vi "Utility Read From Register - Integers.vi"(0 "VISA resource name":refnum<visa-resource-name>, 1 "Unit Address (1)":u8=1, 5 "Register Address (0)":u16, 9 "Num Of Reg (1)":u16=1 min=1 step=1, 11 "error in (no error)":errorcluster) -> (4 "VISA resource name out":refnum<visa-resource-name>, 6 "Data":i16[](array[numeric]), 15 "error out":errorcluster)   [LabVIEW 2010, in "Eurotherm 32xx Series.lvlib"]
doc: "This VI reads value from specified registers of specified unit."
uses:
  <instrlib>/Eurotherm 32xx Series/Eurotherm 32xx Series.lvlib
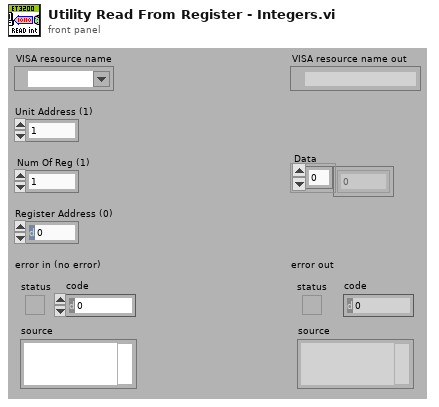
[diagram p1: front panel]
types:
  T1 = cluster{"Read Buffer[0]":u8, "Read Buffer[1]":u8}
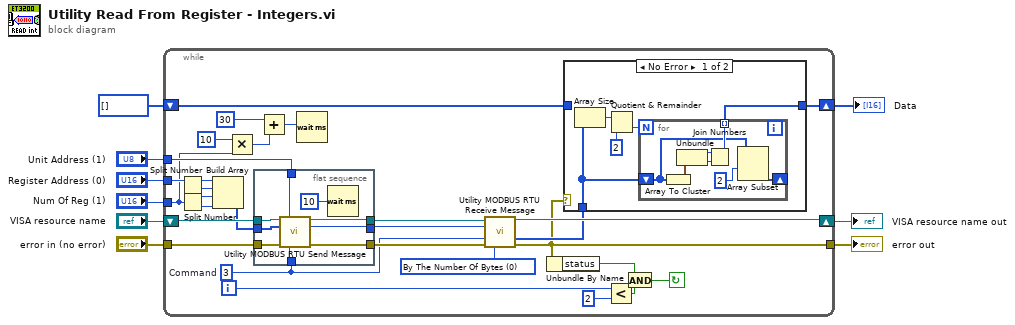
[diagram p0: block diagram]
diagram:
  n1 = while {
    tunnel: "Unit Address (1)" -> [w19]
    shift-right: [w35] -> w8
    shift-left: "VISA resource name" -> [w36]
    tunnel: "Register Address (0)" -> [w25]
    tunnel: "Num Of Reg (1)" -> [w11]
    shift-right: [w23] -> w6
    shift-left: u16[] [] -> [w22]
    tunnel: [w17] -> w2
    tunnel: "error in (no error)" -> [w16]
    i -> [w31]
    stop <- w33 continue-if-true
    w10 = u16 0 items=["By The Number Of Bytes", "Copy Of The Sent Message"] ("Receive Message Type (0: By The Number Of Bytes)")
    w32 = u8 3  # Command
    n2 = Split Number(x=w25) -> (hi(x)=w27:u8, lo(x)=w26:u8)
    n3 = Split Number(x=w11) -> (hi(x)=w21:u8, lo(x)=w20:u8)
    n4 = Build Array(w27, w26, w21, w20) -> (w28:u8[])
    n5 = Multiply(x=u32 10, y=w11) -> (x*y=w14:u32)
    n6 = flat-sequence {
      tunnel: [w47] -> w38
      tunnel: [w46] -> w37
      tunnel: w36 -> [w45]
      tunnel: w32 -> [w44]
      tunnel: w28 -> [w43]
      tunnel: w19 -> [w42]
      tunnel: [w39] -> w18
      tunnel: w16 -> [w41]
      frame #0 {
        n7 = call <instrlib>:"Utility MODBUS RTU Send Message.vi"("VISA resource name"=w45, "Unit Address (1)"=w42, "Message (empty array)"=w43, "error in (no error)"=w41, "Command (0)"=w44) -> ("VISA resource name out"=w46:refnum<visa-resource-name>, "Length Of Sent MSG"=w39:u8, "error out"=w47:errorcluster)  [unwired: 8 in]
        n8 = Wait (ms)(milliseconds to wait=u32 10) -> ()  [unwired: 1 out]
      }
    }
    n9 = Add(x=u32 30 ("milliseconds to wait"), y=w14) -> (x+y=w13:u32)
    n10 = Wait (ms)(milliseconds to wait=w13) -> ()  [unwired: 1 out]
    n11 = call <instrlib>:"Utility MODBUS RTU Receive Message.vi"("VISA resource name"=w37, "Length Of Sent MSG (0)"=w18, "Sent Command (0)"=w32, "error in (no error)"=w38, "Receive Message Type (0: By The Number Of Bytes)"=w10) -> ("VISA resource name out"=w35:refnum<visa-resource-name>, "Read Buffer"=w24:u8[], "error out"=w17:errorcluster)  [unwired: 8 in]
    n12 = Unbundle By Name(w17) -> ("status"=w34:bool)
    n13 = case shown="No Error" w17 {
      tunnel: w24 -> [w52 _]
      tunnel: [w51 w60] -> w23
      tunnel: w22 -> [_ w60]
      frame No Error {
        n14 = Array Size(array=w52) -> (size(s)=w50:i32)
        n15 = Quotient & Remainder(x=w50, y=2) -> (floor(x/y)=w48:i32)  [unwired: 1 out]
        n16 = for {
          N: w48 -> [_]
          shift-right: [w54] -> _
          shift-left: w52 -> [w55]
          tunnel: [w56] -> w51 mode=indexing
          n17 = Array To Cluster(array=w55) -> (cluster=w59:T1)
          n18 = Unbundle(w59) -> ("Read Buffer[0]"=w57:u8, "Read Buffer[1]"=w58:u8)
          n19 = Join Numbers(hi=w57, lo=w58) -> ((hi.lo)=w56:u16)
          n20 = Array Subset(array=w55, index=2) -> (w54:u8[])  [unwired: 1 in]
        }
      }
      frame Error {
      }
    }
    n21 = Less?(x=w31, y=2) -> (x < y?=w30:bool)
    n22 = And(x=w34, y=w30) -> (x .and. y?=w33:bool)
  }
  "error out" <- w2
  "VISA resource name out" <- w8
  "Data" <- w6
